vi "Filter Graphics by Folder Name.vi"(9 "Tag":string, 11 "Glyphs [] in":T1[](array[typedef])) -> (3 "Filtered Glyphs []":T1[](array[typedef]))   [LabVIEW 2020, in "Glyph.lvclass"]
uses:
  Class/Icon Library/Glyph.lvclass
  Controls/Path&Icon.ctl
  vi.lib/LabVIEW Icon API/lv_icon/Controls/Graphic.ctl
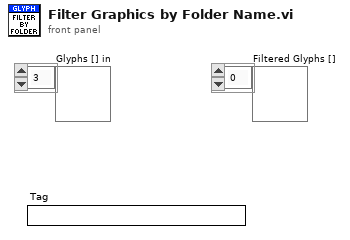
[diagram p1: front panel]
types:
  T1 = typedef "Graphic.ctl" = cluster{"Rectangle":cluster{"left":i16, "top":i16, "right":i16, "bottom":i16}, "Path":path, "Image":picture, "Filter":string, "FileName":string}
  T2 = typedef "Path&Icon.ctl" = cluster{"Rectangle":cluster{"left":i16, "top":i16, "right":i16, "bottom":i16}, "Path":path, "Image":picture, "Filter":string, "FileName":string}
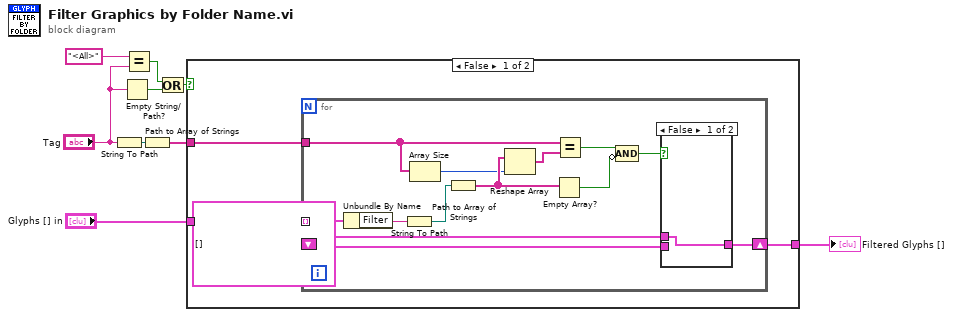
[diagram p0: block diagram]
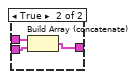
[diagram p2: hidden frame]
diagram:
  n1 = String To Path(string="Tag") -> (path=w1:path)
  n2 = Empty String/Path?(string/path="Tag") -> (empty?=w5:bool)
  n3 = Equal?(x="<All>", y="Tag") -> (x = y?=w6:bool)
  n4 = Path to Array of Strings(0:w1) -> (2:w3:string[])  [unwired: 1 out]
  n5 = Or(x=w6, y=w5) -> (x .or. y?=w4:bool)
  n6 = case shown="False" w4 {
    tunnel: "Glyphs [] in" -> [w13 w30]
    tunnel: [w11 w30] -> w8
    tunnel: w3 -> [w10 _]
    frame False {
      n7 = for {
        shift-right: [w24] -> w11
        shift-left: T2[] [] -> [w25]
        tunnel: w13 -> [w23] mode=indexing
        tunnel: w10 -> [w16]
        n8 = Unbundle By Name(w23) -> ("Filter"=w20:string)
        n9 = String To Path(string=w20) -> (path=w19:path)
        n10 = Array Size(array=w16) -> (size(s)=w15:i32)
        n11 = Path to Array of Strings(0:w19) -> (2:w17:string[])  [unwired: 1 out]
        n12 = Reshape Array(w17, w15) -> (w14:string[])
        n13 = Empty Array?(array=w17) -> (empty?=w22:bool)
        n14 = Equal?(x=w16, y=w14) -> (x = y?=w18:bool)
        n15 = Compound Arithmetic op=AND(w18, invert w22) -> (w21:bool)
        n16 = case shown="False" w21 {
          tunnel: w25 -> [w26 w29]
          tunnel: [w26 w28] -> w24
          tunnel: w23 -> [_ w27]
          frame False {
          }
          frame True {
            n17 = Build Array (concatenate)(w29, w27) -> (w28:T1[])
          }
        }
      }
    }
    frame True {
    }
  }
  "Filtered Glyphs []" <- w8
